vi "Config Dev Cutoff.vi"(8 "error in":errorcluster, 10 "Rolloff Point (3000 Hz)":dbl=3000.0 min=0.0002778 max=4200.0, 11 "VISA resource name":refnum<visa-resource-name>) -> (0 "error out":errorcluster, 3 "VISA resource name out":refnum<visa-resource-name>)   [LabVIEW 2019, in "Andeen-Hagerling 2700(400 firmware).lvlib"]
doc: "Sets the upper limit for the 3 db down cutoff frequency to DCutoff in Hertz."
uses:
  Andeen-Hagerling 2700(400 firmware).lvlib
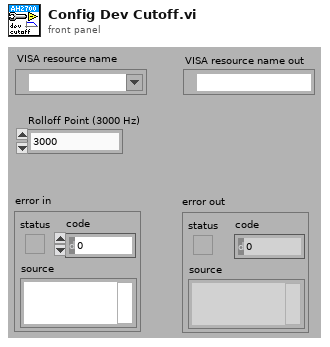
[diagram p1: front panel]
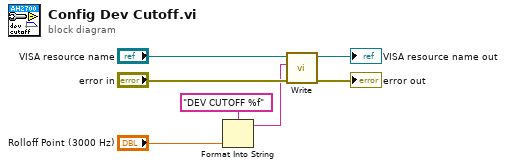
[diagram p0: block diagram]
diagram:
  n1 = Format Into String(format string="DEV CUTOFF %f", "Rolloff Point (3000 Hz)") -> (resulting string=w2:string)  [unwired: 2 in, 1 out]
  n2 = call "Write.vi"("error in"="error in", "command"=w2, "VISA resource name"="VISA resource name") -> ("error out"=→"error out":errorcluster, "VISA resource name out"=→"VISA resource name out":refnum<visa-resource-name>)  [unwired: 7 in]
